vi "encendido_apagado_cluster_led.vi"() -> ()   [LabVIEW 2024]
panel:
  in  "stop":bool
  out "Cluster":cluster{"D1":bool, "D2":bool}
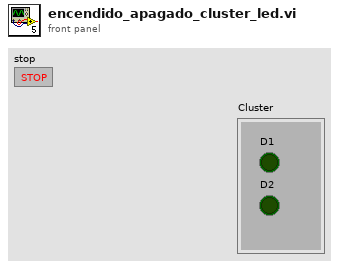
[diagram p1: front panel]
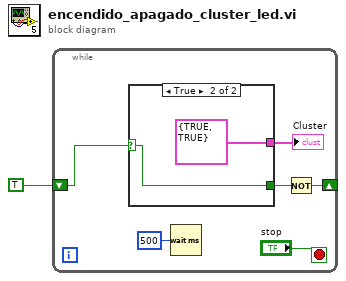
[diagram p0: block diagram]
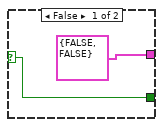
[diagram p2: hidden frame]
diagram:
  n1 = while {
    shift-right: [w5] -> _
    shift-left: TRUE -> [w3]
    stop <- "stop" stop-if-true
    n2 = case shown="True" w3 {
      selector: w3 -> [w8 w10]
      tunnel: [cluster{bool, bool} {FALSE, FALSE} cluster{bool, bool} {TRUE, TRUE}] -> w2
      tunnel: [w8 w10] -> w6
      frame False {
      }
      frame True {
      }
    }
    "Cluster" <- w2
    n3 = Wait (ms)(milliseconds to wait=u32 500) -> ()  [unwired: 1 out]
    n4 = Not(x=w6) -> (.not. x?=w5:bool)
  }
